vi "Get Logging Interface.vi"(11 "Dispatcher Thread in":refnum<class "Dispatcher Thread.lvclass">) -> (2 "Logging Interface":refnum<class "Logging Interface.lvclass">, 3 "Dispatcher Thread out":refnum<class "Dispatcher Thread.lvclass">)   [LabVIEW 2020, in "DSF Core.lvlib" / "Dispatcher Thread.lvclass"]
uses:
  Thread/Dispatcher/Dispatcher Thread.lvclass
  Logging/Logging Interface.lvclass
  Thread/Dispatcher/Dispatcher Thread.lvclass/Dispatcher Thread.ctl
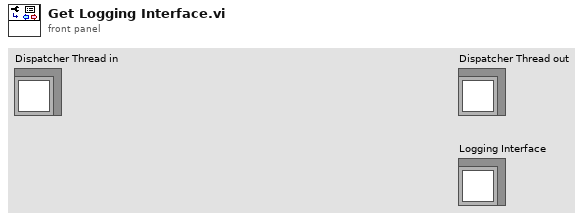
[diagram p1: front panel]
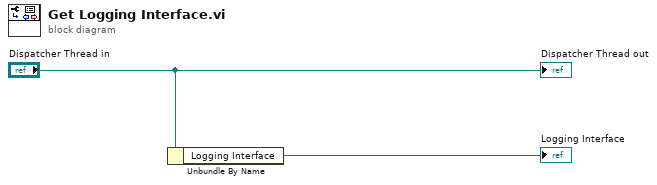
[diagram p0: block diagram]
diagram:
  n1 = Unbundle By Name("Dispatcher Thread in") -> ("Logging Interface"=→"Logging Interface":refnum<class "Logging Interface.lvclass">)
  "Dispatcher Thread out" <- "Dispatcher Thread in"
